vi "ricalcola con nuovo file taratura.vi"(6 "Densità per ricalcolo P2":dbl, 8 "rpm nom":dbl, 9 "Coefficenti P2":T1, 10 "Indici":T2, 11 "dati in":string[][](array[string])) -> (3 "dati out":string[][](array[string]))   [LabVIEW 2019]
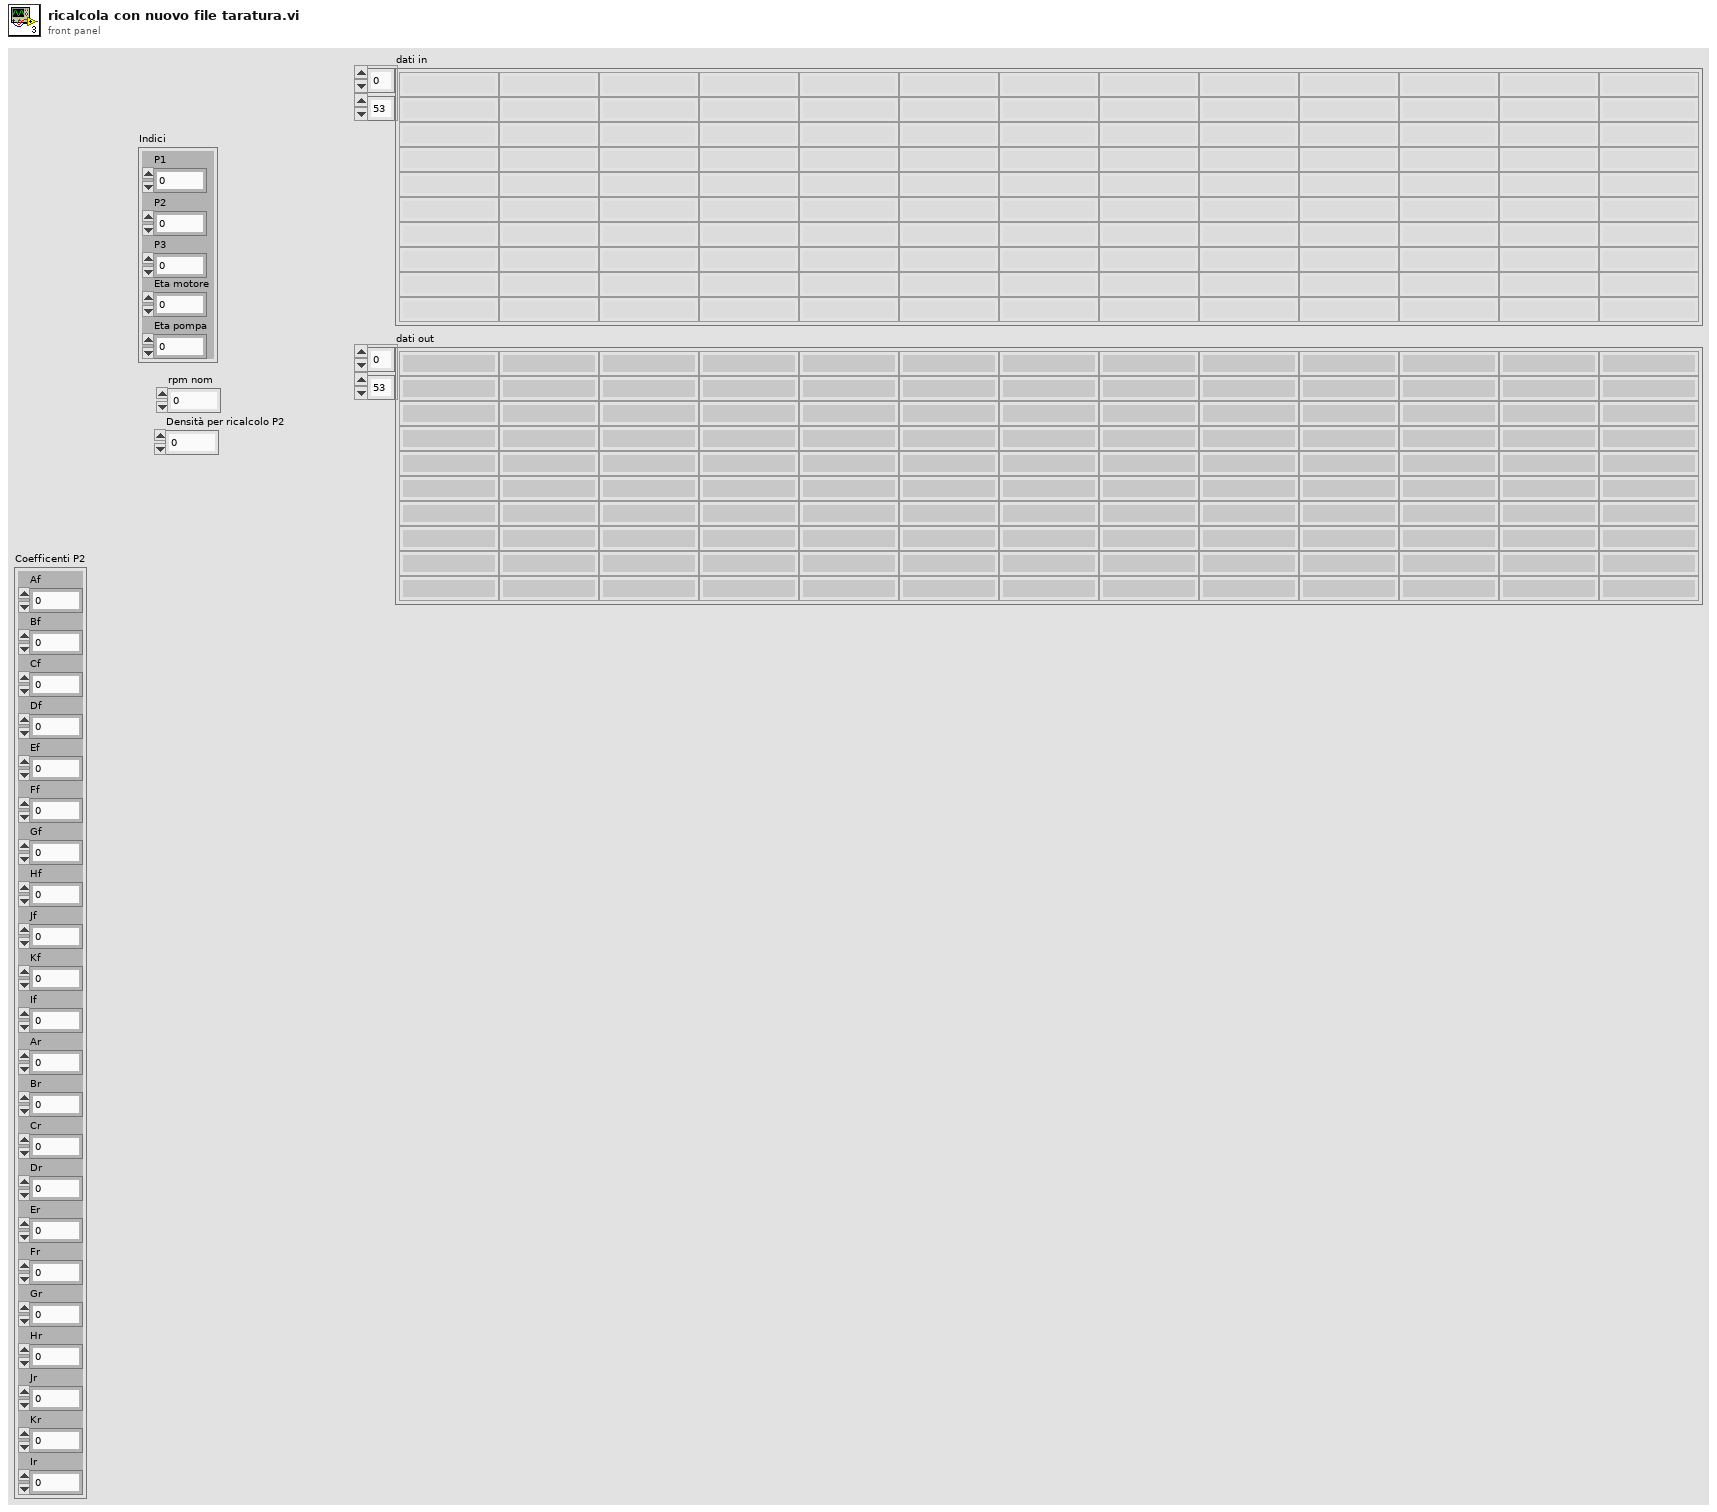
[diagram p1: front panel]
types:
  T1 = cluster{"Af":dbl, "Bf":dbl, "Cf":dbl, "Df":dbl, "Ef":dbl, "Ff":dbl, "Gf":dbl, "Hf":dbl, "Jf":dbl, "Kf":dbl, "If":dbl, "Ar":dbl, "Br":dbl, "Cr":dbl, "Dr":dbl, "Er":dbl, "Fr":dbl, "Gr":dbl, "Hr":dbl, "Jr":dbl, "Kr":dbl, "Ir":dbl}
  T2 = cluster{"P1":i32, "P2":i32, "P3":i32, "Eta motore":i32, "Eta pompa":i32}
  T3 = enum32{"Torsiometro", "coeff p2", "Rendimento", "Curva rend"}
  T4 = cluster{"dati in[0]":string, "dati in[1]":string, "dati in[2]":string, "dati in[3]":string, "dati in[4]":string, "dati in[5]":string, "dati in[6]":string, "dati in[7]":string, "dati in[8]":string, "dati in[9]":string, "dati in[10]":string, "dati in[11]":string, "dati in[12]":string, "dati in[13]":string, "dati in[14]":string, "dati in[15]":string, "dati in[16]":string, "dati in[17]":string, "dati in[18]":string, "dati in[19]":string, "dati in[20]":string, "dati in[21]":string, "dati in[22]":string, "dati in[23]":string, "dati in[24]":string, "dati in[25]":string, "dati in[26]":string, "dati in[27]":string, "dati in[28]":string, "dati in[29]":string, "dati in[30]":string, "dati in[31]":string, "dati in[32]":string, "dati in[33]":string, "dati in[34]":string, "dati in[35]":string, "dati in[36]":string, "dati in[37]":string, "dati in[38]":string, "dati in[39]":string, "dati in[40]":string, "dati in[41]":string, "dati in[42]":string, "dati in[43]":string, "dati in[44]":string, "dati in[45]":string, "dati in[46]":string, "dati in[47]":string, "dati in[48]":string, "dati in[49]":string, "dati in[50]":string, "dati in[51]":string, "dati in[52]":string, "dati in[53]":string, "dati in[54]":string, "dati in[55]":string, "dati in[56]":string, "dati in[57]":string, "dati in[58]":string, "dati in[59]":string, "dati in[60]":string, "dati in[61]":string, "dati in[62]":string, "dati in[63]":string, "dati in[64]":string, "dati in[65]":string, "dati in[66]":string, "dati in[67]":string, "dati in[68]":string, "dati in[69]":string, "dati in[70]":string, "dati in[71]":string, "dati in[72]":string, "dati in[73]":string, "dati in[74]":string, "dati in[75]":string, "dati in[76]":string, "dati in[77]":string, "dati in[78]":string, "dati in[79]":string, "dati in[80]":string, "dati in[81]":string, "dati in[82]":string, "dati in[83]":string, "dati in[84]":string, "dati in[85]":string, "dati in[86]":string, "dati in[87]":string, "dati in[88]":string, "dati in[89]":string, "dati in[90]":string, "dati in[91]":string, "dati in[92]":string, "dati in[93]":string, "dati in[94]":string, "dati in[95]":string, "dati in[96]":string, "dati in[97]":string, "dati in[98]":string, "dati in[99]":string, "dati in[100]":string, "dati in[101]":string, "dati in[102]":string, "dati in[103]":string, "dati in[104]":string, "dati in[105]":string, "dati in[106]":string, "dati in[107]":string, "dati in[108]":string, "dati in[109]":string, "dati in[110]":string}
  T5 = typedef "MISURE NM.ctl" = cluster{"Banco":string, "Anno":string, "Numero":string, "Ntabella":string, "Misura":string, "Tipo Prova":string, "ProgressivoAcq":string, "Descrizione":string, "Data_ora":string, "t. acq [h:m:s]":string, "t. acq [min]":string, "t. acq [s]":string, "n [rpm]":string, "f [Hz]":string, "U1[V]":string, "U2 [V]":string, "U3 [V]":string, "U123_media [V]":string, "I1[A]":string, "I2[A]":string, "I3[A]":string, "I123_media [A]*I":string, "I_123_sbil [%]":string, "Ulin[V]":string, "Uc [V]":string, "Uaux [V]":string, "Ilin[A]*I":string, "Imar[A]":string, "Iaux[A]":string, "Uarm[V]":string, "Uecc[V]":string, "Iarm[A]*I":string, "Iecc[A]":string, "pf":string, "P1 [W]":string, "P1 [kW]":string, "Q [VAR]":string, "Q [kVAR]":string, "S [VA]":string, "S [kVA]":string, "P1arm[W]":string, "P1ecc[W]":string, "Parm[kW]":string, "P1ecc[kW]":string, "Cond[uF]":string, "P1_linea_6fili[W]":string, "P1_linea_6fili[kW]":string, "eta_gr_6fili [%]":string, "eta_inverter_6fili [%]":string, "pf_linea_6fili":string, "U4 [V]":string, "U5 [V]":string, "U6 [V]":string, "U456_media [V]":string, "I4 [A]":string, "I5 [A]":string, "I6 [A]":string, "I456_media [A]":string, "C [Nm]*C":string, "Cric [Nm]":string, "Cric\\Cnom":string, "Iric[A]":string, "Iric\\Inom":string, "P2_mecc [W]":string, "P2_mecc [kW]":string, "eta motore [%]":string, "Scorr[%]":string, "Tamb[°C]":string, "R1[ohm]":string, "R2[ohm]":string, "R3[ohm]":string, "Rmedia[ohm]":string, "DT_R1[°C]":string, "DT_R2[°C]":string, "DT_R3[°C]":string, "DT_media[°C]":string, "R_marcia[ohm]":string, "R_aux[ohm]":string, "DT_marcia[°C]":string, "DT_aux[°C]":string, "R_Arm[ohm]":string, "R_Ecc[ohm]":string, "DT_Arm[°C]":string, "DT_Ecc[°C]":string, "TambFreddo[°C]":string, "R1_freddo[ohm]":string, "R2_freddo[ohm]":string, "R3_freddo[ohm]":string, "Rmedia_freddo[ohm]":string, "R_Marcia_freddo[ohm]":string, "R_Aux_freddo[ohm]":string, "R_Arm_freddo[ohm]":string, "R_Ecc_freddo[ohm]":string, "TC1 [°C]":string, "TC2 [°C]":string, "TC3 [°C]":string, "TC4 [°C]":string, "TC5 [°C]":string, "TC6 [°C]":string, "TC7 [°C]":string, "TC8 [°C]":string, "PT1000_1[°C]":string, "PT1000_2[°C]":string, "PT1000_3[°C]":string, "Vdc eccitatrice[V]":string, "Idc eccitatrice[A]":string, "Vdc rotore[V]":string, "Idc rotore[A]":string, "Vac rotore[V]":string, "Iac rotore[V]":string, "V dinamo[V]":string, "Portata Q":string, "Pressione H":string, "U1'[V]":string, "U2'[V]":string, "U3'[V]":string, "I1'[A]":string, "I2'[A]":string, "I3'[A]":string, "U''R-N":string, "U''S-N":string, "U'' T-N":string, "U''R-S":string, "U''R-T":string, "U''S-T":string, "I1''[A]":string, "I2''[A]":string, "I3''[A]":string, "F''[Hz]":string, "P''[kW]":string, "CosFi''":string, "PT1000_4[°C]":string, "Scorta 3":string}
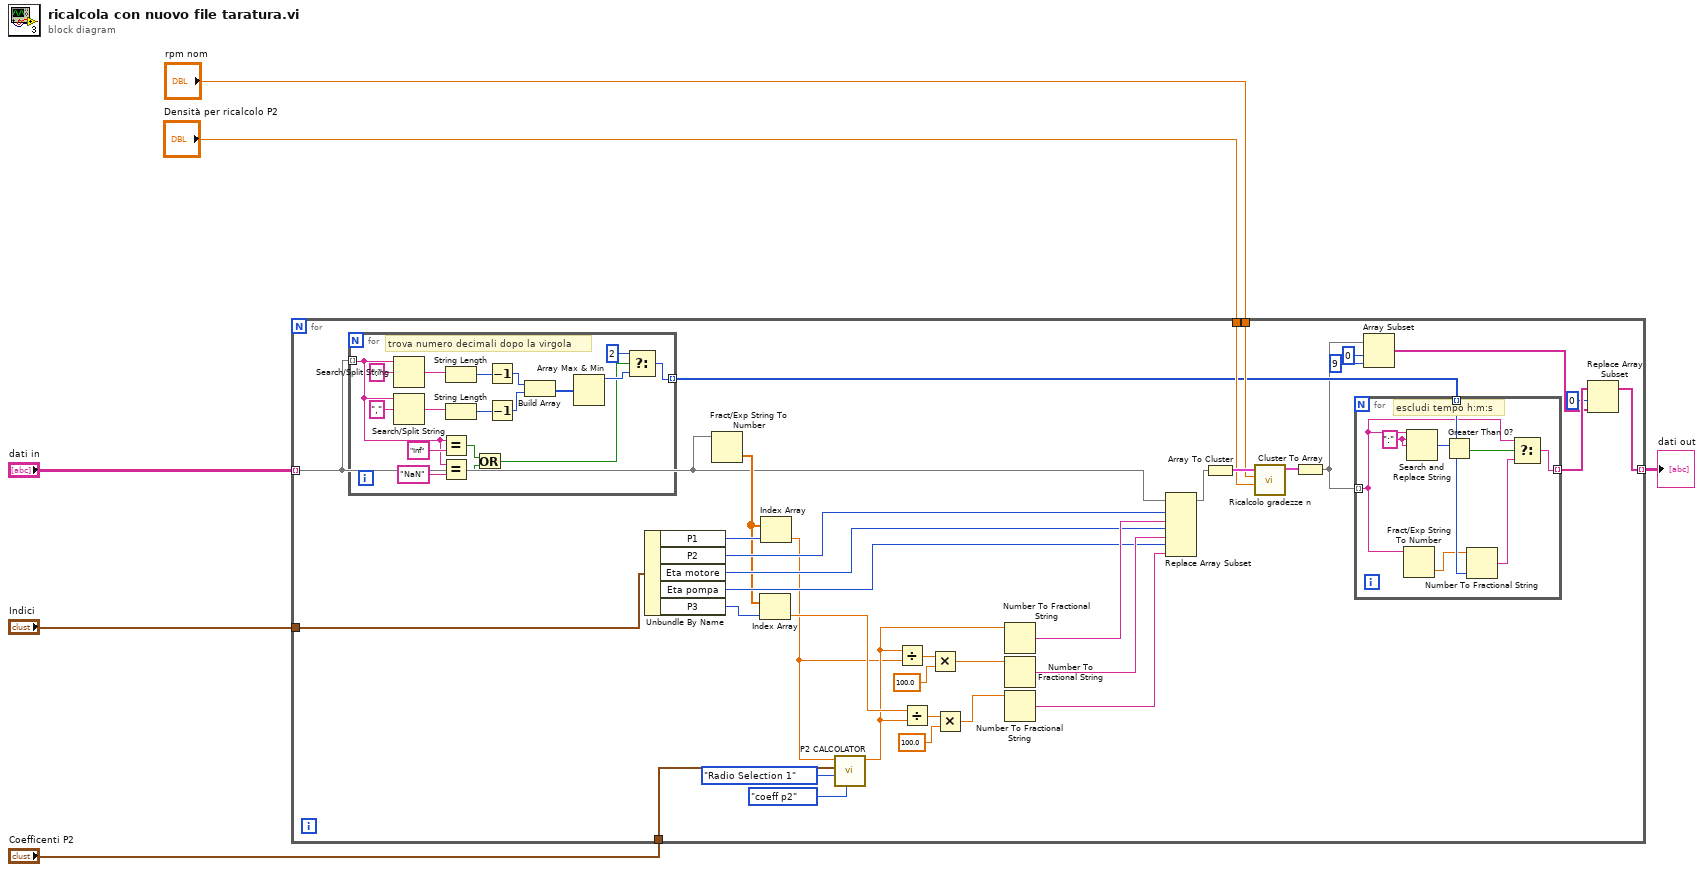
[diagram p0: block diagram]
diagram:
  n1 = for {
    tunnel: "dati in" -> [w17] mode=indexing
    tunnel: "Coefficenti P2" -> [w40]
    tunnel: [w7] -> w5 mode=indexing
    tunnel: "Indici" -> [w39]
    tunnel: "rpm nom" -> [w19]
    tunnel: "Densità per ricalcolo P2" -> [w18]
    n2 = for {
      tunnel: w17 -> [w49] mode=indexing
      tunnel: [w45] -> w16 mode=indexing
      # "trova numero decimali dopo la virgola"
      n3 = Search/Split String(string=w49, search string/char (-)=".") -> (match + rest of string=w60:string)  [unwired: 1 in, 2 out]
      n4 = Search/Split String(string=w49, search string/char (-)=",") -> (match + rest of string=w55:string)  [unwired: 1 in, 2 out]
      n5 = Equal?(x=w49, y="Inf") -> (x = y?=w50:bool)
      n6 = Equal?(x=w49, y="NaN") -> (x = y?=w47:bool)
      n7 = String Length(string=w60) -> (length=w59:i32)
      n8 = String Length(string=w55) -> (length=w56:i32)
      n9 = Or(x=w50, y=w47) -> (x .or. y?=w44:bool)
      n10 = Decrement(x=w59) -> (x-1=w54:i32)
      n11 = Decrement(x=w56) -> (x-1=w53:i32)
      n12 = Build Array(w54, w53) -> (w52:i32[])
      n13 = Array Max & Min(array=w52) -> (max value=w46:i32)  [unwired: 3 out]
      n14 = Select(t=2, s=w44, f=w46) -> (s? t:f=w45:i32)
    }
    n15 = Unbundle By Name(w39) -> ("P1"=w38:i32, "P2"=w37:i32, "Eta motore"=w32:i32, "Eta pompa"=w27:i32, "P3"=w25:i32)
    n16 = Fract/Exp String To Number(string=w17) -> (number=w26:dbl[])  [unwired: 3 in, 1 out]
    n17 = Index Array(array=w26, index=w25) -> (element=w22:dbl)
    n18 = Index Array(array=w26, index=w38) -> (element=w14:dbl)
    n19 = call "P2 CALCOLATOR.vi"("Calcolo P2"=T3."coeff p2", "Coefficienti P2"=enum32{"Radio Selection 1", "Radio Selection 2"}."Radio Selection 1", "Coefficenti P2"=w40, "P1  kw"=w14) -> ("P2"=w15:dbl)  [unwired: 7 in]
    n20 = Divide(x=w15, y=w14) -> (x/y=w31:dbl)
    n21 = Divide(x=w22, y=w15) -> (x/y=w23:dbl)
    n22 = Multiply(x=w31, y=100.0) -> (x*y=w29:dbl)
    n23 = Multiply(x=w23, y=100.0) -> (x*y=w21:dbl)
    n24 = Number To Fractional String(number=w15) -> (F-format string=w36:string)  [unwired: 3 in]
    n25 = Number To Fractional String(number=w29) -> (F-format string=w28:string)  [unwired: 3 in]
    n26 = Number To Fractional String(number=w21) -> (F-format string=w20:string)  [unwired: 3 in]
    n27 = Replace Array Subset(array=w17, new element #1=w36, index #1=w37, new element #2=w28, index #2=w32, new element #3=w20, index #3=w27) -> (w33:string[])
    n28 = Array To Cluster(array=w33) -> (cluster=w35:T4)
    n29 = call "Ricalcolo gradezze n.vi"("Densità per ricalcolo P2"=w18, "rpm nom"=w19, "MISURE NM in"=w35) -> ("MISURE NM out"=w34:T5)  [unwired: 8 in]
    n30 = Cluster To Array(cluster=w34) -> (array=w12:string[])
    n31 = for {
      tunnel: w12 -> [w61] mode=indexing
      tunnel: w16 -> [w68] mode=indexing
      tunnel: [w62] -> w13 mode=indexing
      w66 = ":" ("search string")
      # "escludi tempo h:m:s"
      n32 = Fract/Exp String To Number(string=w61) -> (number=w67:dbl)  [unwired: 3 in, 1 out]
      n33 = Search and Replace String(input string=w61, search string=w66, replace string=w66) -> (number of replacements=w65:i32)  [unwired: 5 in, 3 out]
      n34 = Greater Than 0?(x=w65) -> (x > 0?=w64:bool)
      n35 = Number To Fractional String(number=w67, precision (6)=w68) -> (F-format string=w63:string)  [unwired: 2 in]
      n36 = Select(t=w61, s=w64, f=w63) -> (s? t:f=w62:string)
    }
    n37 = Array Subset(array=w12, index=0, length=9) -> (w8:string[])
    n38 = Replace Array Subset(array=w13, new element=w8, index=0) -> (w7:string[])
  }
  "dati out" <- w5
